vi "ajouterdonneepointage.vi"(0 "Heure":string caption="heure", 1 "Identifiant":dbl, 2 "Fichier DB":string) -> ()   [LabVIEW 2024]
uses:
  <vilib>/drjdpowell/SQLite Library/SQL Connection/Connection.lvclass
  <vilib>/drjdpowell/SQLite Library/SQL Connection/Open (string).vi
  <vilib>/drjdpowell/SQLite Library/SQLite.lvlib
  <vilib>/drjdpowell/SQLite Library/SQL Connection/Execute SQL (No results).vi
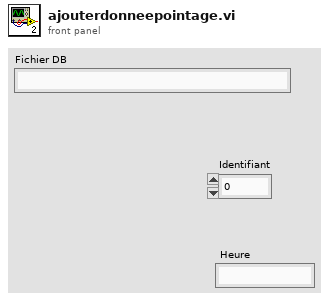
[diagram p1: front panel]
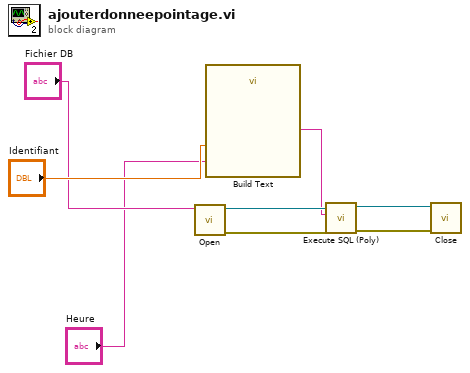
[diagram p0: block diagram]
diagram:
  n1 = call-poly <vilib>:"Open.vi"("db file"="Fichier DB") -> ("error out"=w7:errorcluster, "SQLite Connection"=w8:refnum<class "Connection.lvclass">)  [unwired: 9 in]
  n2 = call "Build Text"("id"="Identifiant", "heure"="Heure") -> ("Result"=w6:string)  [unwired: 12 in, 1 out]
  n3 = call-poly <vilib>:"Execute SQL (Poly).vi"("error in (no error)"=w7, "SQL"=w6, "SQLite Connection in"=w8) -> ("error out"=w4:errorcluster, "SQLite Connection"=w3:refnum<class "Connection.lvclass">)  [unwired: 7 in]
  n4 = call-dynamic "Close.vi"("error in (no error)"=w4, "SQLite Connection in"=w3) -> ()  [unwired: 9 in, 1 out]
